vi "rqcBob SPD State Viewer.vi"() -> ()   [LabVIEW 2018]
uses:
  hidSPDLibForLabView/LibVIs/hidSPD Controls/hidSPD Viwer State.ctl
  hidSPDLibForLabView/LibVIs/hidSPD Controls/hidSPD Device Session.ctl
  hidSPDLibForLabView/hidSPDLibForLabView.lvlib
panel:
  out "SPD2 Heatsink T":sgl(graph) caption="Heatsink T"
  out "SPD2 Diod T":sgl(graph) caption="Diod T"
  out "SPD2 Ready":bool caption="Ready"
  out "error out":errorcluster
  in  "Stop":bool
  out "SPD1 Heatsink T":sgl(graph) caption="Heatsink T"
  out "SPD1 Diod T":sgl(graph) caption="Diod T"
  out "SPD1 Ready":bool caption="Ready"
  # "SPD1"
  # "SPD2"
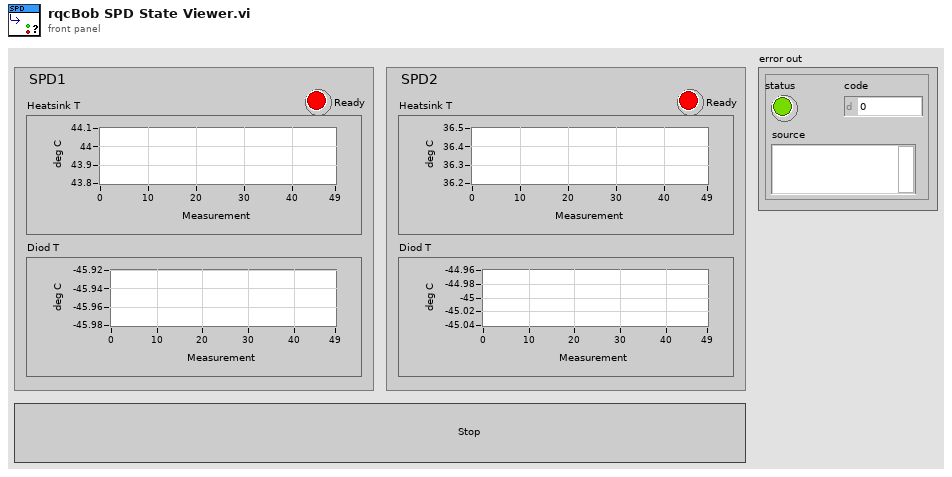
[diagram p1: front panel]
types:
  T1 = typedef "hidSPDLibForLabView.lvlib/hidSPD Device Session.ctl" = cluster{"spdDevicePointer":u64}
  T2 = typedef "hidSPDLibForLabView.lvlib/hidSPD Viwer State.ctl" = enum16{"open sessions", "close sessions", "read reports"}
  T3 = typedef "hidSPDLibForLabView.lvlib/hidSPD HidDevInfo.ctl" = cluster{"name":string, "path":string}
  T4 = typedef "hidSPDLibForLabView.lvlib/hidSPD Simple Report.ctl" = cluster{"Heatsink Temprature":sgl, "Diod Temprature":sgl, "TEC-voltage":sgl, "Diod Bias":sgl, "RF Power":sgl, "Thermal used":sgl, "hv bias used":sgl, "hv code used":u16, "strobe code used":u16, "SPD number":u8, "SPD ready":u8}
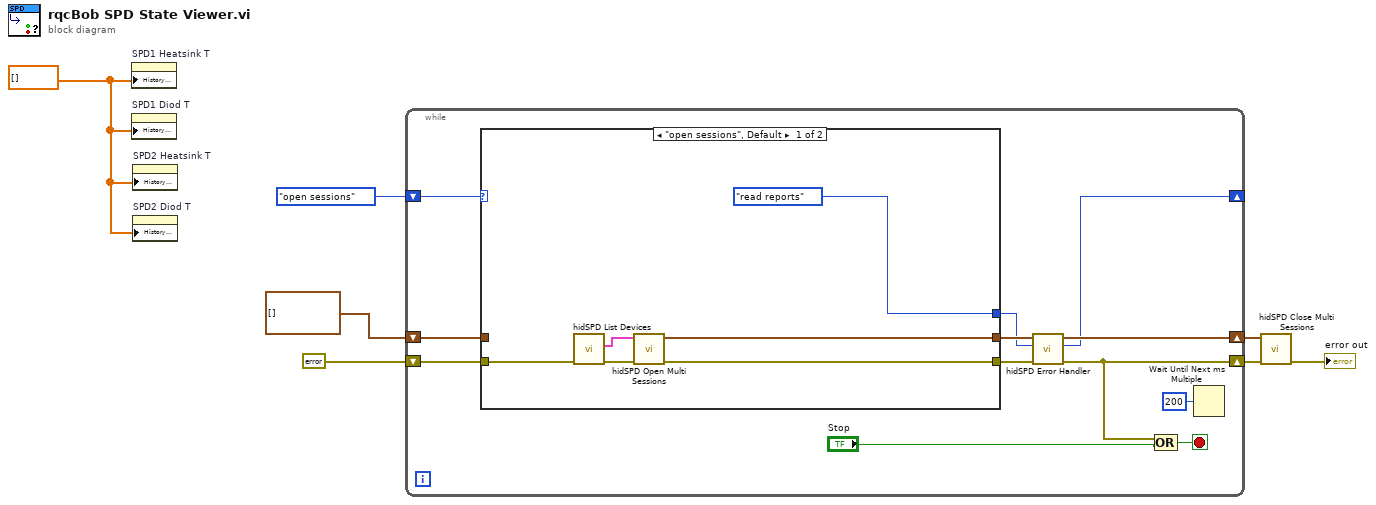
[diagram p0: block diagram]
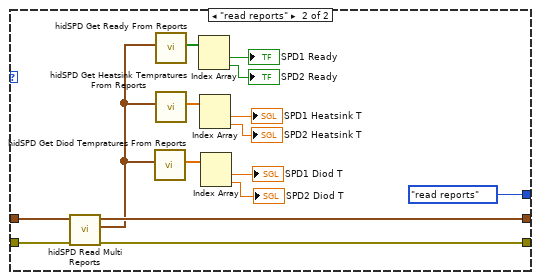
[diagram p2: hidden frame]
diagram:
  w4 = sgl[] [] ("History Data")
  n1 = property on="SPD1 Heatsink T" class="WFChart (strict)"("History Data"=w4) -> ()  [unwired: 2 in, 2 out]
  n2 = property on="SPD1 Diod T" class="WFChart (strict)"("History Data"=w4) -> ()  [unwired: 2 in, 2 out]
  n3 = property on="SPD2 Heatsink T" class="WFChart (strict)"("History Data"=w4) -> ()  [unwired: 2 in, 2 out]
  n4 = property on="SPD2 Diod T" class="WFChart (strict)"("History Data"=w4) -> ()  [unwired: 2 in, 2 out]
  n5 = while {
    shift-right: [w12] -> w6
    shift-left: T1[] [] ("spdDevSessions out") -> [w19]
    shift-right: [w10] -> w5
    shift-left: errorcluster {"status"=FALSE, "code"=0, "source"=""} ("error in (no error)") -> [w18]
    shift-right: [w8] -> _
    shift-left: hidSPD_Viwer_State."open sessions" ("hidSPD Viewer State") -> [w14]
    stop <- w16 stop-if-true
    n6 = case shown="\"open sessions\", Default" w14 {
      tunnel: w19 -> [_ w40]
      tunnel: w18 -> [w21 w39]
      tunnel: [w23 w38] -> w13
      tunnel: [w22 w37] -> w11
      tunnel: [hidSPD_Viwer_State."read reports" ("hidSPD Viewer State") hidSPD_Viwer_State."read reports" ("hidSPD Viewer State")] -> w9
      frame "open sessions", Default {
        n7 = call "hidSPD List Devices.vi"("error in (no error)"=w21) -> ("error out"=w25:errorcluster, "devices list"=w24:T3[])  [unwired: 9 in]
        n8 = call "hidSPD Open Multi Sessions.vi"("error in (no error)"=w25, "devices list"=w24) -> ("error out"=w22:errorcluster, "spdDevSessions out"=w23:T1[])  [unwired: 8 in]
      }
      frame "read reports" {
        n9 = call "hidSPD Read Multi Reports.vi"("error in (no error)"=w39, "spdDevSessions in"=w40) -> ("error out"=w37:errorcluster, "spd Reports"=w36:T4[], "spdDevSessions out"=w38:T1[])  [unwired: 7 in]
        n10 = call "hidSPD Get Diod Tempratures From Reports.vi"("spd Reports in"=w36) -> ("Diod Tempratures"=w33:sgl[])  [unwired: 10 in]
        n11 = call "hidSPD Get Ready From Reports.vi"("spd Reports in"=w36) -> ("Ready"=w31:bool[])  [unwired: 10 in]
        n12 = call "hidSPD Get Heatsink Tempratures From Reports.vi"("spd Reports in"=w36) -> ("Heatsink Tempratures"=w35:sgl[])  [unwired: 10 in]
        n13 = Index Array(array=w31) -> (element #1=→"SPD1 Ready":bool, element #2=→"SPD2 Ready":bool)  [unwired: 2 in]
        n14 = Index Array(array=w35) -> (element #1=→"SPD1 Heatsink T":sgl, element #2=→"SPD2 Heatsink T":sgl)  [unwired: 2 in]
        n15 = Index Array(array=w33) -> (element #1=→"SPD1 Diod T":sgl, element #2=→"SPD2 Diod T":sgl)  [unwired: 2 in]
      }
    }
    n16 = call "hidSPD Error Handler.vi"("error in (no error)"=w11, "hidSPD Viewer State in"=w9, "spdDevSessions in"=w13) -> ("error out"=w10:errorcluster, "hidSPD Viewer State out"=w8:T2, "spdDevSessions out"=w12:T1[])  [unwired: 6 in]
    n17 = Compound Arithmetic op=OR(w10, "Stop") -> (w16:bool)
    n18 = Wait Until Next ms Multiple(millisecond multiple=u32 200) -> ()  [unwired: 1 out]
  }
  n19 = call "hidSPD Close Multi Sessions.vi"("error in (no error)"=w5, "spdDevSessions out"=w6) -> ("error out"=→"error out":errorcluster)  [unwired: 9 in]
